vi "Display Frame.vi"(8 "Error In":errorcluster, 10 "Frame":u32[][](array[colorbox]), 11 "Display In":refnum<class "Neopixel - Host.lvclass">) -> (0 "Error Out":errorcluster, 3 "Display Out":refnum<class "Neopixel - Host.lvclass">)   [LabVIEW 2021, in "Neopixel - Host.lvclass"]
uses:
  Neopixel - Host.lvclass
  Neopixel - Host.lvclass/Neopixel - Host.ctl
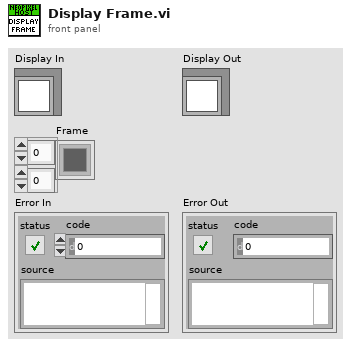
[diagram p1: front panel]
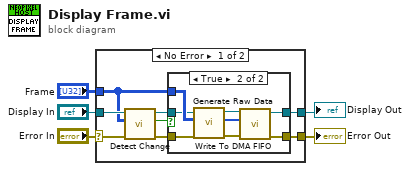
[diagram p0: block diagram]
diagram:
  n1 = case shown="No Error" "Error In" {
    selector: "Error In" -> [w10 w24]
    tunnel: "Display In" -> [w11 w25]
    tunnel: [w13 w24] -> w3
    tunnel: [w12 w25] -> w2
    tunnel: "Frame" -> [w9 _]
    frame No Error {
      n2 = call "Detect Change.vi"("Error In"=w10, "Frame"=w9, "Display In"=w11) -> ("Error Out"=w8:errorcluster, "Frame Change"=w7:bool, "Display Out"=w6:refnum<class "Neopixel - Host.lvclass">)  [unwired: 6 in]
      n3 = case shown="True" w7 {
        tunnel: [w14 w23] -> w13
        tunnel: [w15 w22] -> w12
        tunnel: w9 -> [_ w18]
        tunnel: w8 -> [w14 w17]
        tunnel: w6 -> [w15 w16]
        frame False {
        }
        frame True {
          n4 = call "Generate Raw Data.vi"("Error In"=w17, "Matrix"=w18, "Display In"=w16) -> ("Error Out"=w20:errorcluster, "Raw Data"=w19:u8[], "Display Out"=w21:refnum<class "Neopixel - Host.lvclass">)  [unwired: 6 in]
          n5 = call "Write To DMA FIFO.vi"("Error In"=w20, "Data"=w19, "Display In"=w21) -> ("Error Out"=w23:errorcluster, "Display Out"=w22:refnum<class "Neopixel - Host.lvclass">)  [unwired: 7 in]
        }
      }
    }
    frame Error {
    }
  }
  "Error Out" <- w3
  "Display Out" <- w2
